vi "PhotonTrackedTarget_Unpack.vi"(9 "StartByte":i32, 11 "RawData":u8[](array[numeric])) -> (1 "NextByte":i32, 3 "TrackedTarget":T1={"Yaw"=0.0, "Pitch"=0.0, "Area"=0.0, "Skew"=0.0, "MinAreaRectCorners"=[], "BestCameraToTarget"={"TRANSLATION3D"={"X"=0.0, "Y"=0.0, "Z"=0.0}, "ROTATION3D"={"Q_quaternion"={"R"=1.0, "V"=[0.0, 0.0, 0.0]}}, "XF"=FALSE}, "FiducialId"=0, "AltCameraToTarget"={"TRANSLATION3D"={"X"=0.0, "Y"=0.0, "Z"=0.0}, "ROTATION3D"={"Q_quaternion"={"R"=1.0, "V"=[0.0, 0.0, 0.0]}}, "XF"=FALSE}, "PoseAmbiguity"=0.0, "DetectedCorners"=[], "ObjDetectId"=0, "ObjDetectConf"=0.0} {"AltCameraToTarget"."TRANSLATION3D"."Z" format="%14.3f"; "AltCameraToTarget"."TRANSLATION3D"."Y" format="%14.3f"; "AltCameraToTarget"."TRANSLATION3D"."X" format="%14.3f"; "BestCameraToTarget"."TRANSLATION3D"."Z" format="%14.3f"; "BestCameraToTarget"."TRANSLATION3D"."Y" format="%14.3f"; "BestCameraToTarget"."TRANSLATION3D"."X" format="%14.3f"})   [LabVIEW 2019, in "PhotonVisionLib.lvlib"]
doc: "Internal function to parse the data for each target returned by PhotonCamera_GetLatestResult.\n\nInputs:\n - RawData -- Byte array containing the data to parse.\n\nOutputs:\n - TrackedTarget -- Parsed TrackedTarget cluster."
uses:
  PhotonVisionLib.lvlib
  TypeDef/PhotonTrackedTargetType.ctl
  TypeDef/TargetCornerType.ctl
  <vilib>/Rock Robotics/WPI/ThirdParty/JAS_Junk/TrajLib/TypeDef/TRANSFORM3D.ctl
  <vilib>/Rock Robotics/WPI/ThirdParty/JAS_Junk/TrajLib/TypeDef/TRANSLATION3D.ctl
  <vilib>/Rock Robotics/WPI/ThirdParty/JAS_Junk/TrajLib/TypeDef/ROTATION3D.ctl
  <vilib>/Rock Robotics/WPI/ThirdParty/JAS_Junk/TrajLib/TypeDef/QUATERNION.ctl
  <vilib>/Rock Robotics/WPI/ThirdParty/JAS_Junk/TrajLib/VI/Transform3d_Create_Trans3dRot3d.vi
  <vilib>/Rock Robotics/WPI/ThirdParty/JAS_Junk/TrajLib/VI/Translation3d_Create.vi
  <vilib>/Rock Robotics/WPI/ThirdParty/JAS_Junk/TrajLib/VI/Rotation3d_Create_Quaternion.vi
  <vilib>/Rock Robotics/WPI/ThirdParty/JAS_Junk/TrajLib/VI/Quaternion_New.vi
  <vilib>/Rock Robotics/WPI/ThirdParty/JAS_Junk/TrajLib/VI/Quaternion_Normalize.vi
  <vilib>/Rock Robotics/WPI/ThirdParty/JAS_Junk/TrajLib/VI/Quaternion_New_Default.vi
  <vilib>/Rock Robotics/WPI/ThirdParty/JAS_Junk/TrajLib/Trajectory_Library.lvlib
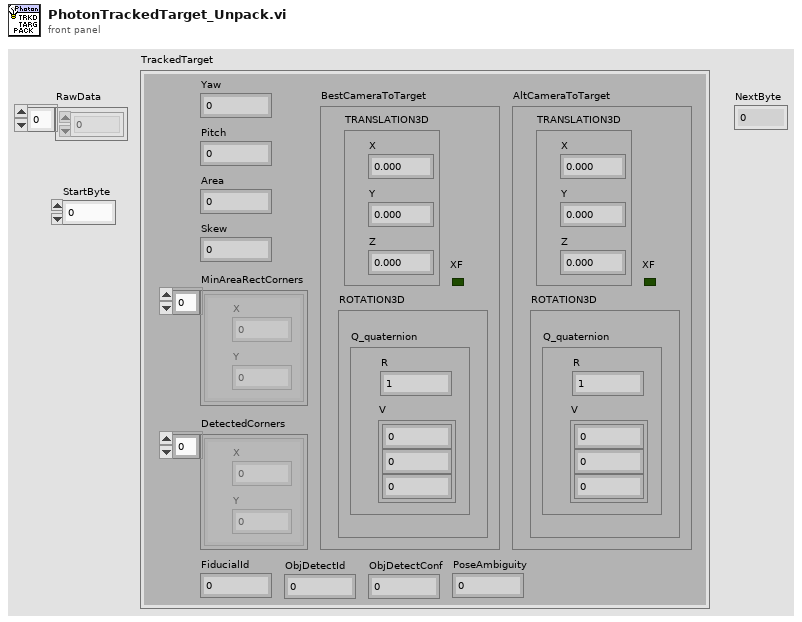
[diagram p1: front panel]
types:
  T1 = typedef "PhotonVisionLib.lvlib/PhotonTrackedTargetType.ctl" = cluster{"Yaw":dbl, "Pitch":dbl, "Area":dbl, "Skew":dbl, "MinAreaRectCorners":T2[], "BestCameraToTarget":T3, "FiducialId":i32, "AltCameraToTarget":T3, "PoseAmbiguity":dbl, "DetectedCorners":T2[], "ObjDetectId":i32, "ObjDetectConf":sgl}
  T2 = typedef "PhotonVisionLib.lvlib/TargetCornerType.ctl" = cluster{"X":dbl, "Y":dbl}
  T3 = typedef "Trajectory_Library.lvlib/TRANSFORM3D.ctl" = cluster{"TRANSLATION3D":T4, "ROTATION3D":T5, "XF":bool}
  T4 = typedef "Trajectory_Library.lvlib/TRANSLATION3D.ctl" = cluster{"X":dbl, "Y":dbl, "Z":dbl}
  T5 = typedef "Trajectory_Library.lvlib/ROTATION3D.ctl" = cluster{"Q_quaternion":T6}
  T6 = typedef "Trajectory_Library.lvlib/QUATERNION.ctl" = cluster{"R":dbl, "V":dbl[]}
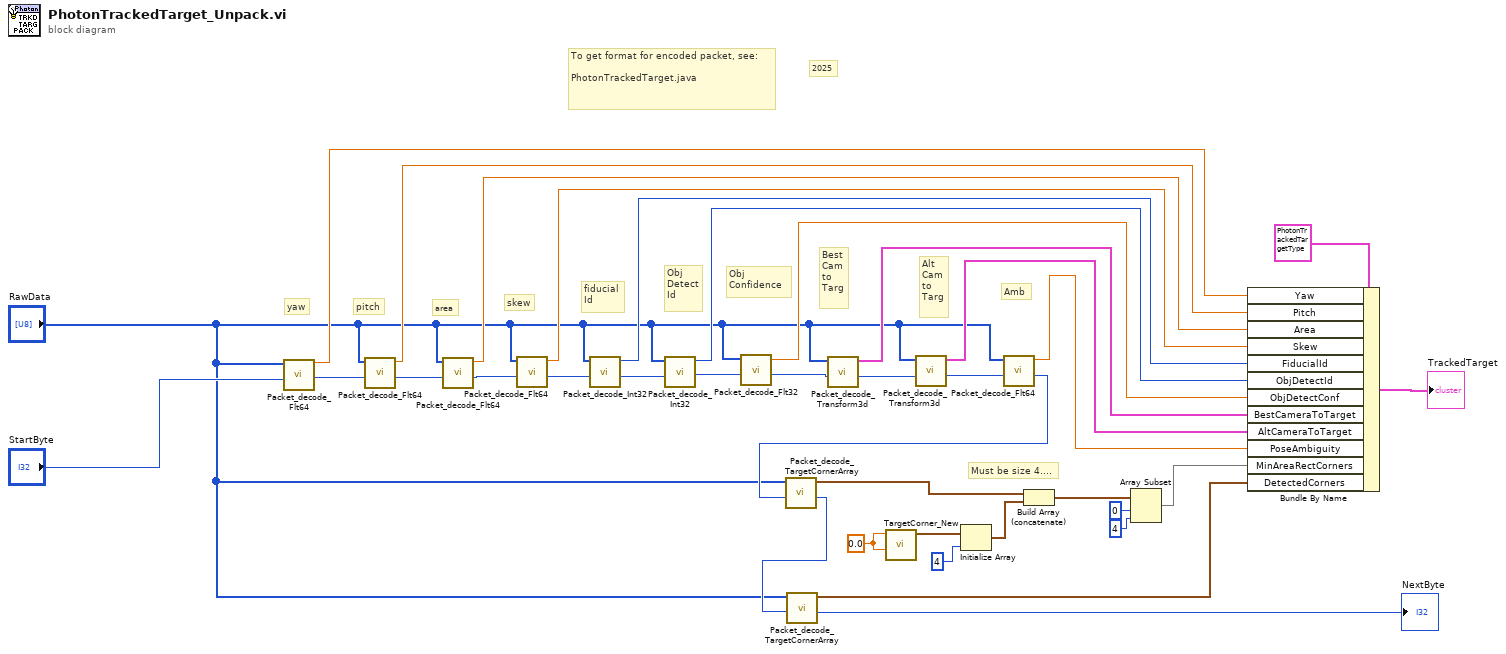
[diagram p0: block diagram]
diagram:
  w12 = 0.0 ("X")
  # "Must be size 4...."
  # "Obj\nConfidence"
  # "Obj\nDetect\nId"
  # "2025"
  # "To get format for encoded packet, see:\n\nPhotonTrackedTarget.java"
  # "Amb"
  # "Alt\nCam\nto\nTarg"
  # "Best\nCam\nto\nTarg"
  # "fiducial\nId"
  # "skew"
  # "area"
  # "pitch"
  # "yaw"
  n1 = call "Packet_decode_Flt64.vi"("StartByte"="StartByte", "RawData"="RawData") -> ("NextByte"=w33:i32, "Flt64_Value"=w36:dbl)  [unwired: 8 in]
  n2 = call "Packet_decode_Flt64.vi"("StartByte"=w33, "RawData"="RawData") -> ("NextByte"=w31:i32, "Flt64_Value"=w32:dbl)  [unwired: 8 in]
  n3 = call "Packet_decode_Flt64.vi"("StartByte"=w31, "RawData"="RawData") -> ("NextByte"=w28:i32, "Flt64_Value"=w30:dbl)  [unwired: 8 in]
  n4 = call "Packet_decode_Flt64.vi"("StartByte"=w28, "RawData"="RawData") -> ("NextByte"=w26:i32, "Flt64_Value"=w27:dbl)  [unwired: 8 in]
  n5 = call "Packet_decode_Int32.vi"("StartByte"=w26, "RawData"="RawData") -> ("NextByte"=w19:i32, "Int32_Value"=w25:i32)  [unwired: 8 in]
  n6 = call "Packet_decode_Int32.vi"("StartByte"=w19, "RawData"="RawData") -> ("NextByte"=w17:i32, "Int32_Value"=w18:i32)  [unwired: 8 in]
  n7 = call "Packet_decode_Flt32.vi"("StartByte"=w17, "RawData"="RawData") -> ("NextByte"=w16:i32, "Flt32_Value"=w15:sgl)  [unwired: 8 in]
  n8 = call "Packet_decode_Transform3d.vi"("NextByte in"=w16, "RawData"="RawData") -> ("NextByte out"=w23:i32, "Transform3d"=w24:T3)  [unwired: 6 in]
  n9 = call "TargetCorner_New.vi"("Y"=w12, "X"=w12) -> ("TargetCorner"=w14:T2)  [unwired: 9 in]
  n10 = call "Packet_decode_Transform3d.vi"("NextByte in"=w23, "RawData"="RawData") -> ("NextByte out"=w21:i32, "Transform3d"=w22:T3)  [unwired: 6 in]
  n11 = Initialize Array(w14, 4 ("dimension size")) -> (w10:T2[])
  n12 = call "Packet_decode_Flt64.vi"("StartByte"=w21, "RawData"="RawData") -> ("NextByte"=w5:i32, "Flt64_Value"=w20:dbl)  [unwired: 8 in]
  n13 = call "Packet_decode_TargetCornerArray.vi"("NextByte in"=w5, "RawData"="RawData") -> ("NextByte out"=w4:i32, "TargetCornerArray"=w11:T2[])  [unwired: 6 in]
  n14 = call "Packet_decode_TargetCornerArray.vi"("NextByte in"=w4, "RawData"="RawData") -> ("NextByte out"=→"NextByte":i32, "TargetCornerArray"=w2:T2[])  [unwired: 6 in]
  n15 = Build Array (concatenate)(w11, w10) -> (w9:T2[])
  n16 = Array Subset(array=w9, index=0, length=4) -> (w6:T2[])
  n17 = Bundle By Name(cluster=T1 {"Yaw"=0.0, "Pitch"=0.0, "Area"=0.0, "Skew"=0.0, "MinAreaRectCorners"=[], "BestCameraToTarget"={"TRANSLATION3D"={"X"=0.0, "Y"=0.0, "Z"=0.0}, "ROTATION3D"={"Q_quaternion"={"R"=1.0, "V"=[0.0, 0.0, 0.0]}}, "XF"=FALSE}, "FiducialId"=0, "AltCameraToTarget"={"TRANSLATION3D"={"X"=0.0, "Y"=0.0, "Z"=0.0}, "ROTATION3D"={"Q_quaternion"={"R"=1.0, "V"=[0.0, 0.0, 0.0]}}, "XF"=FALSE}, "PoseAmbiguity"=0.0, "DetectedCorners"=[], "ObjDetectId"=0, "ObjDetectConf"=0.0} ("PhotonTrackedTarget"), "Yaw"=w36, "Pitch"=w32, "Area"=w30, "Skew"=w27, "FiducialId"=w25, "ObjDetectId"=w18, "ObjDetectConf"=w15, "BestCameraToTarget"=w24, "AltCameraToTarget"=w22, "PoseAmbiguity"=w20, "MinAreaRectCorners"=w6, "DetectedCorners"=w2) -> (→"TrackedTarget":T1)
